vi "manual_controller.vi"() -> ()   [LabVIEW 2012]
uses:
  MagiQmw3.lvclass
panel:
  out "Total errors":i32
  out "Errors":errorcluster[](array[cluster])
  out "Updates":i32=6
  in  "Slot":u16=4 max=10
  in  "Clock type":enum8{"Internal", "External", "PXI"}(ring)
  in  "ch2 enable":bool
  in  "Ch2 freq":dbl=100.0 caption="Frequency (MHz)" min=25.0 max=6000.0
  in  "Ch2 atten":i32(slide) min=0 max=10 step=1 scale=0.01..10.0
  in  "ch1 enable":bool
  in  "Ch1 freq":dbl=8000.0 caption="Frequency (MHz)" min=7300.0 max=8200.0
  in  "Ch1 atten":i32(slide) min=0 max=10 step=1 scale=0.01..10.0
  in  "stop":bool
  in  "ch0 enable":bool
  in  "Ch0 freq":dbl=100.0 caption="Frequency (MHz)" min=25.0 max=6000.0
  in  "Ch0 atten":i32(slide) min=0 max=10 step=1 scale=0.01..10.0
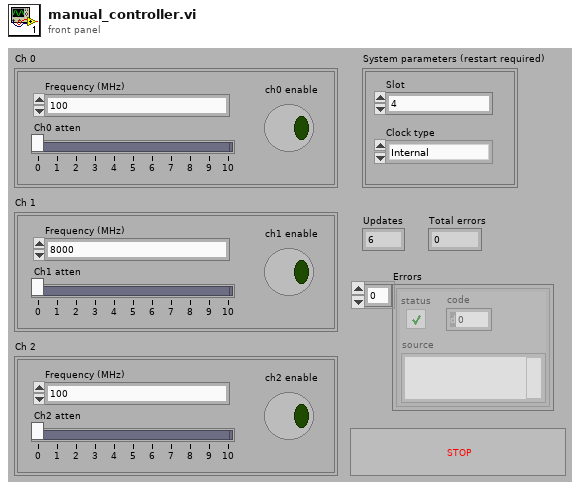
[diagram p1: front panel]
types:
  T1 = cluster{"ch0 enable":bool, "Ch0 freq":dbl, "Ch0 atten":i32}
  T2 = cluster{"ch1 enable":bool, "Ch1 freq":dbl, "Ch1 atten":i32}
  T3 = cluster{"ch2 enable":bool, "Ch2 freq":dbl, "Ch2 atten":i32}
  T4 = cluster{"ch2 enable":bool, "Ch2 freq":dbl, "Ch2 atten":i32}[]
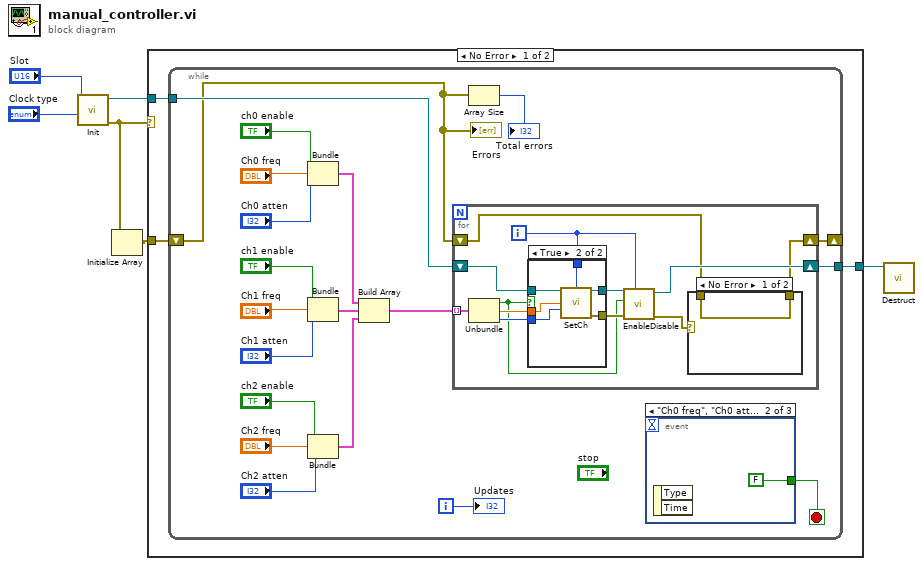
[diagram p0: block diagram]
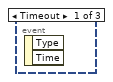
[diagram p2: hidden frame]
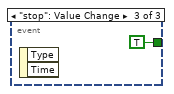
[diagram p3: hidden frame]
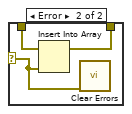
[diagram p4: hidden frame]
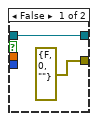
[diagram p5: hidden frame]
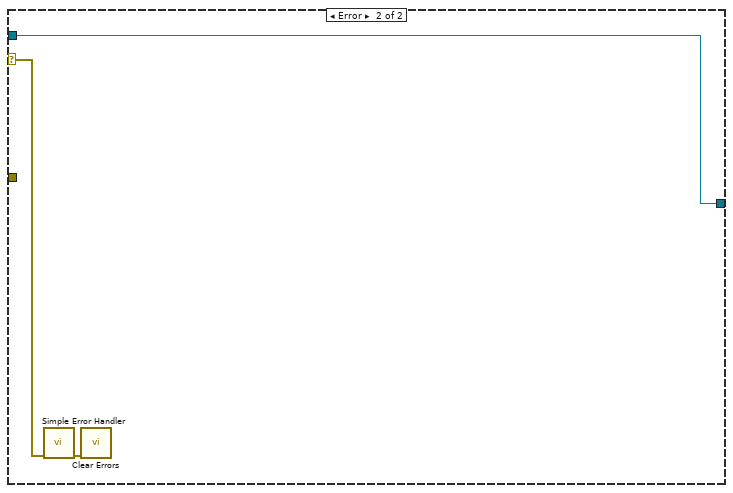
[diagram p6: hidden frame]
diagram:
  n1 = call "Init.vi"("Clock type"="Clock type", "Slot"="Slot") -> ("error out"=w2:errorcluster, "MagiQmw3 out"=w6:refnum<class "MagiQmw3.lvclass">)  [unwired: 8 in]
  n2 = Initialize Array(w2) -> (w1:errorcluster[])  [unwired: 1 in]
  n3 = case shown="No Error" w2 {
    selector: w2 -> [_ w57]
    tunnel: w6 -> [w9 w56]
    tunnel: [w8 w56] -> w3
    tunnel: w1 -> [w7 _]
    frame No Error {
      n4 = while {
        tunnel: w9 -> [w15]
        tunnel: [w16] -> w8
        shift-right: [w13] -> _
        shift-left: w7 -> [w12]
        i -> [w14]
        stop <- w10 stop-if-true
        n5 = Bundle("ch0 enable"="ch0 enable", "Ch0 freq"="Ch0 freq", "Ch0 atten"="Ch0 atten") -> (w20:T1)  [unwired: 1 in]
        n6 = Bundle("ch1 enable"="ch1 enable", "Ch1 freq"="Ch1 freq", "Ch1 atten"="Ch1 atten") -> (w19:T2)  [unwired: 1 in]
        n7 = Bundle("ch2 enable"="ch2 enable", "Ch2 freq"="Ch2 freq", "Ch2 atten"="Ch2 atten") -> (w18:T3)  [unwired: 1 in]
        n8 = Build Array(w20, w19, w18) -> (w17:T4)
        n9 = for {
          tunnel: w17 -> [w43] mode=indexing
          shift-right: [w37] -> w16
          shift-left: w15 -> [w36]
          shift-right: [w33] -> w13
          shift-left: w12 -> [w34]
          i -> [w40]
          n10 = Unbundle(w43) -> ("ch2 enable"=w35:bool, "Ch2 freq"=w42:dbl, "Ch2 atten"=w41:i32)
          n11 = case shown="True" w35 {
            tunnel: [w49 w55] -> w39
            tunnel: [errorcluster {"status"=FALSE, "code"=0, "source"=""} ("error out") w54] -> w38
            tunnel: w42 -> [_ w53]
            tunnel: w41 -> [_ w52]
            tunnel: w40 -> [_ w51]
            tunnel: w36 -> [w49 w50]
            frame False {
            }
            frame True {
              n12 = call "SetCh.vi"("MagiQmw3 in"=w50, "ch"=w51, "freq"=w53, "atten"=w52) -> ("MagiQmw3 out"=w55:refnum<class "MagiQmw3.lvclass">, "error out"=w54:errorcluster)  [unwired: 10 in]
            }
          }
          n13 = call "EnableDisable.vi"("ch"=w40, "error in (no error)"=w38, "Enable"=w35, "MagiQmw3 in"=w39) -> ("error out"=w32:errorcluster, "MagiQmw3 out"=w37:refnum<class "MagiQmw3.lvclass">)  [unwired: 6 in]
          n14 = case shown="No Error" w32 {
            selector: w32 -> [_ w45]
            tunnel: w34 -> [w44 w47]
            tunnel: [w44 w46] -> w33
            frame No Error {
            }
            frame Error {
              n15 = Insert Into Array(array=w47, new element=w45) -> (w46:errorcluster[])  [unwired: 1 in]
              n16 = call <vilib>:"Clear Errors.vi"("error in (no error)"=w45) -> ()  [unwired: 6 in, 1 out]
            }
          }
        }
        n17 = Array Size(array=w12) -> (size(s)=→"Total errors":i32)
        n18 = event shown="[1] \"Ch0 freq\", \"Ch0 atten\", \"ch0 enable\", \"Ch1 atten\", \"Ch1 freq\", \"ch1 enable\", \"Ch2 atten\", \"Ch2 freq\", \"ch2 enable\": Value Change" {
          selector: _ -> [_ _ _]
          dyn-events: _ -> [_ _ _]
          timeout: _ -> [_ _ _]
          tunnel: [_ FALSE TRUE] -> w10
          event Timeout {
            n19 = event-data() -> ()  [unwired: 1 in, 2 out]
          }
          event "Ch0 freq", "Ch0 atten", "ch0 enable", "Ch1 atten", "Ch1 freq", "ch1 enable", "Ch2 atten", "Ch2 freq", "ch2 enable": Value Change {
            n20 = event-data() -> ()  [unwired: 1 in, 2 out]
          }
          event "stop": Value Change {
            n21 = event-data() -> ()  [unwired: 1 in, 2 out]
          }
        }
        "Updates" <- w14
        "Errors" <- w12
      }
    }
    frame Error {
      n22 = call <vilib>:"Simple Error Handler.vi"("error in (no error)"=w57) -> ("error out"=w58:errorcluster)  [unwired: 4 in, 4 out]
      n23 = call <vilib>:"Clear Errors.vi"("error in (no error)"=w58) -> ()  [unwired: 6 in, 1 out]
    }
  }
  n24 = call "Destruct.vi"("MagiQmw3 in"=w3) -> ()  [unwired: 10 in, 1 out]
